vi "Actor Core.vi"(8 "error in":errorcluster, 11 "RandomDataChart in":refnum<class "MultiSubscriber.lvclass">) -> (0 "error out":errorcluster, 3 "Actor out":refnum<class "Actor.lvclass">)   [LabVIEW 2018, in "TestViewables.lvlib" / "MultiSubscriber.lvclass"]
doc: "(<B>Filename</B>: Actor Framework.lvlib:Actor.lvclass:Actor Core.vi)\n\nReceives messages to the actor, reacts to them, and initiates any error handling that may shut the actor down.\n\nDescendant classes may override this VI to append parallel tasks for the actor to complete while it handles messages. Overrides use the Call Parent Method node.\n\n<License>\nCopyright © 2017 Composed Systems, LLC | All rights reserved\nwww.composed.io\n\nAuthor: Ethan Stern <ethan.stern@composed.io>\n\nThis software is provided \"AS IS\" WITHOUT WARRANTIES, either express or implied, AND IS FOR EDUCATIONAL PURPOSES ONLY.\n</License>"
uses:
  MultiSubscriber.lvclass
  <vilib>/ActorFramework/Actor/Actor.lvclass
  MultiSubscriber Messages/Notification Msg/UpdateChart Msg.lvclass
  <vilib>/event_ctls.llb/lveventtype.ctl
  modules/mva-core/Source/SubscriptionPolicy/BasicSubscription/BasicSubscription.lvclass/BasicSubscription.ctl
  <vilib>/ActorFramework/Actor/Actor.lvclass/Actor.ctl
  <vilib>/ActorFramework/Message Enqueuer/Message Enqueuer.lvclass/Message Enqueuer.ctl
  modules/composed-transport/Source/Concrete/ActorMessageTransport/ActorMessageTransport.lvclass/ActorMessageTransport.ctl
  modules/mva-core/Source/IMediator/SubscriptionRequest/SubscriptionRequest.lvclass/SubscriptionRequest.ctl
  modules/mva-core/Source/IObserver/IObserver Messages/Subscribe Msg/Subscribe Msg.lvclass/Subscribe Msg.ctl
  MultiSubscriber.lvclass/MultiSubscriber.ctl
  modules/mva-core/Source/IMediator/SubscriptionRequest/Pack Subscription Request.vi
  modules/mva-core/Source/IObserver/IObserver Messages/Subscribe Msg/Send Subscribe.vi
  <vilib>/ActorFramework/Actor/Read Self Enqueuer.vi
  modules/composed-transport/Source/Concrete/ActorMessageTransport/Construct Actor Message Transport.vi
  <vilib>/ActorFramework/Message Enqueuer/Enqueue.vi
  <vilib>/ActorFramework/Message Enqueuer/Init from Existing Queue.vi
  <vilib>/ActorFramework/Message Enqueuer/Equals Not A Refnum.vi
  modules/mva-core/Source/SubscriptionPolicy/BasicSubscription/BasicSubscription.lvclass
  modules/mva-core/Source/IObserver/IObserver/IObserver.lvclass
  C:/Program Files (x86)/National Instruments/LabVIEW 2018/vi.lib/ActorFramework/Actor/Actor.lvclass
  modules/composed-transport/Source/Concrete/ActorMessageTransport/ActorMessageTransport.lvclass
  modules/mva-core/Source/IObserver/IObserver Messages/Subscribe Msg/Subscribe Msg.lvclass
  C:/Program Files (x86)/National Instruments/LabVIEW 2018/vi.lib/ActorFramework/Message/Message.lvclass
  <vilib>/Utility/error.llb/Error Cluster From Error Code.vi
  modules/mva-core/Source/IMediator/ISubscriptionPolicy/Open Subscription Policy.vi
  <vilib>/ActorFramework/Message Priority Queue/Priority Enqueue.vi
  <vilib>/ActorFramework/Message Enqueuer/Message Enqueuer.lvclass
  modules/mva-core/Source/IMediator/SubscriptionRequest/SubscriptionRequest.lvclass
  modules/composed-transport/Source/Concrete/ActorMessageTransport/Notification Msg/Notification Msg.lvclass
  modules/mva-viewable/Source/IViewable/IViewable/IViewable.lvclass
  modules/mva-viewable/Source/ActorEvents/IEventAggregator/IEventAggregator.lvclass
panel:
  in  "Process State":dbl
  in  "Launch Dialog":bool
  out "Cluster":T1
  in  "Random Number":dbl
  out "User Value":dbl(graph)
  # "Black Pane\nif Transparency\nis not working\nproperly"
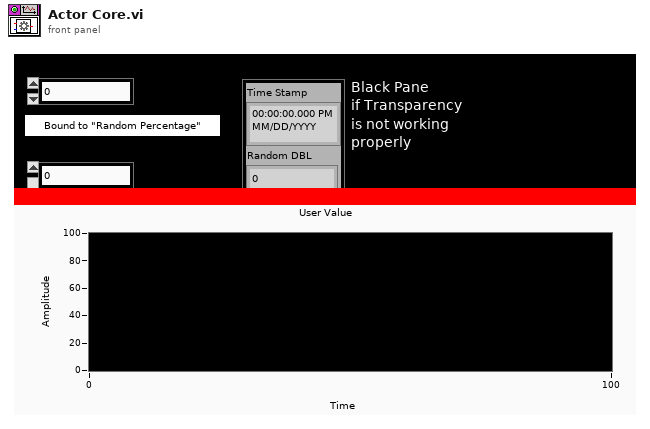
[diagram p1: front panel]
types:
  T1 = cluster{"Time Stamp":timestamp, "Random DBL":dbl}
  T2 = typedef "lveventtype.ctl" = enum32{"Null", "Timeout", "Annotation Menu Selection", "Annotation Menu Selection?", "App Instance Close", "App Instance Close?", "Autoscale Range Change", "Bookmark Info Change", "Cell Edit", "Cell Edit?", "Cursor Grab", "Cursor Grab?", "Cursor Menu Selection", "Cursor Menu Selection?", "Cursor Move", "Cursor Release", "Data Change", "Direction Change", "Display State Change", "Drag Ended", "Drag Enter", "Drag Leave", "Drag Over", "Drag Source Update", "Drag Starting", "Drag Starting?", "Drop", "Exec State Change", "Key Down", "Key Down?", "Key Repeat", "Key Repeat?", "Key Up", "Listbox Double Click", "Menu Activation?", "Menu Selection (App)", "Menu Selection? (App)", "Menu Selection (User)", "Mouse Down", "Mouse Down?", "Mouse Enter", "Mouse Leave", "Mouse Move", "Mouse Up", "Mouse Wheel", "NI Security User Change (App)", "Pane Size", "Panel Close", "Panel Close?", "Panel Resize", "Plot Attribute Change", "Scale Range Change", "Shortcut Menu Activation?", "Shortcut Menu Selection (App)", "Shortcut Menu Selection? (App)", "Shortcut Menu Selection (User)", "Tree Double Click", "Tree Drag", "Tree Drag?", "Tree Drop", "Tree Drop?", "Tree Item Close", "Tree Item Close?", "Tree Item Open", "Tree Item Open?", "User Event", "Value Change"}
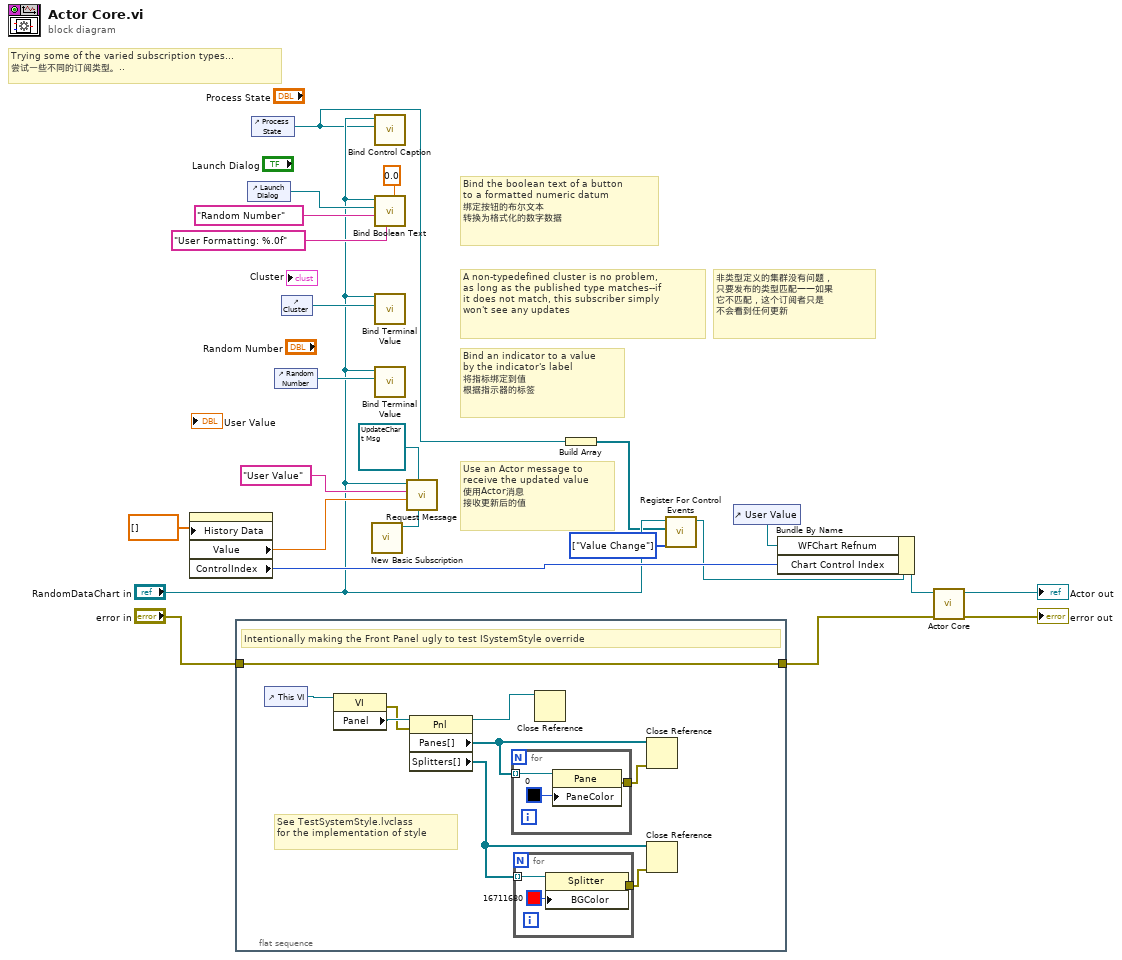
[diagram p0: block diagram]
diagram:
  w1 = T2[] [enum."Value Change"] items=["Null", "Timeout", "Annotation Menu Selection", "Annotation Menu Selection?", "App Instance Close", "App Instance Close?", "Autoscale Range Change", "Bookmark Info Change", "Cell Edit", "Cell Edit?", "Cursor Grab", "Cursor Grab?", "Cursor Menu Selection", "Cursor Menu Selection?", "Cursor Move", "Cursor Release", "Data Change", "Direction Change", "Display State Change", "Drag Ended", "Drag Enter", "Drag Leave", "Drag Over", "Drag Source Update", "Drag Starting", "Drag Starting?", "Drop", "Exec State Change", "Key Down", "Key Down?", "Key Repeat", "Key Repeat?", "Key Up", "Listbox Double Click", "Menu Activation?", "Menu Selection (App)", "Menu Selection? (App)", "Menu Selection (User)", "Mouse Down", "Mouse Down?", "Mouse Enter", "Mouse Leave", "Mouse Move", "Mouse Up", "Mouse Wheel", "NI Security User Change (App)", "Pane Size", "Panel Close", "Panel Close?", "Panel Resize", "Plot Attribute Change", "Scale Range Change", "Shortcut Menu Activation?", "Shortcut Menu Selection (App)", "Shortcut Menu Selection? (App)", "Shortcut Menu Selection (User)", "Tree Double Click", "Tree Drag", "Tree Drag?", "Tree Drop", "Tree Drop?", "Tree Item Close", "Tree Item Close?", "Tree Item Open", "Tree Item Open?", "User Event", "Value Change"] ("Registration Types")
  # "非类型定义的集群没有问题，\n只要发布的类型匹配——如果\n它不匹配，这个订阅者只是\n不会看到任何更新"
  # "Trying some of the varied subscription types...\n尝试一些不同的订阅类型。.."
  # "Bind an indicator to a value\nby the indicator's label\n将指标绑定到值\n根据指示器的标签"
  # "Bind the boolean text of a button\nto a formatted numeric datum\n绑定按钮的布尔文本\n转换为格式化的数字数据"
  # "A non-typedefined cluster is no problem,\nas long as the published type matches--if\nit does not match, this subscriber simply\nwon't see any updates"
  # "Use an Actor message to\nreceive the updated value\n使用Actor消息\n接收更新后的值"
  n1 = property on="User Value" class="WFChart (严格)"("History Data"=dbl[] []) -> ("Value"=w6:dbl, "ControlIndex"=w19:i32)  [unwired: 2 in, 2 out]
  n2 = flat-sequence {
    tunnel: "error in" -> [w26]
    tunnel: [w26] -> w8
    frame #0 {
      # "See TestSystemStyle.lvclass\nfor the implementation of style"
      # "Intentionally making the Front Panel ugly to test ISystemStyle override"
      n3 = control-ref of="This VI"() -> (w32:refnum<vi>)
      n4 = property class="VI"(reference=w32) -> (error out=w24:errorcluster, "Panel"=w31:refnum<vi>)  [unwired: 1 in, 1 out]
      n5 = property class="Pnl"(reference=w31, error in=w24) -> (reference out=w25:refnum<vi>, "Panes[]"=w28:refnum<vi>[], "Splitters[]"=w27:refnum<vi>[])  [unwired: 1 out]
      n6 = for {
        tunnel: [w37] -> w30
        tunnel: w28 -> [w36] mode=indexing
        n7 = property class="Pane"(reference=w36, "PaneColor"=u32 0) -> (error out=w37:errorcluster)  [unwired: 1 in, 1 out]
      }
      n8 = for {
        tunnel: [w34] -> w29
        tunnel: w27 -> [w33] mode=indexing
        n9 = property class="Splitter"(reference=w33, "BGColor"=u32 16711680) -> (error out=w34:errorcluster)  [unwired: 1 in, 1 out]
      }
      n10 = Close Reference(reference=w25) -> ()  [unwired: 1 in, 1 out]
      n11 = Close Reference(reference=w28, error in (no error)=w30) -> ()  [unwired: 1 out]
      n12 = Close Reference(reference=w27, error in (no error)=w29) -> ()  [unwired: 1 out]
    }
  }
  n13 = control-ref of="Launch Dialog"() -> (w10:refnum<vi>)
  n14 = control-ref of="Process State"() -> (w3:refnum<vi>)
  n15 = control-ref of="Random Number"() -> (w21:refnum<vi>)
  n16 = control-ref of="Cluster"() -> (w11:refnum<vi>)
  n17 = call "New Basic Subscription.vi"() -> ("BasicSubscription Out"=w7:refnum<class "BasicSubscription.lvclass">)  [unwired: 11 in]
  n18 = call "Bind Control Caption.vi"("Control Refnum"=w3, "IViewable in"="RandomDataChart in") -> ()  [unwired: 8 in, 2 out]
  n19 = call "Bind Boolean Text.vi"("Datum Type"=0.0, "Format String"="User Formatting: %.0f", "Datum Name (\"\"=Use Control Label)"="Random Number" ("Topic Name (Use Control Text)"), "Bool Refnum"=w10, "IViewable in"="RandomDataChart in") -> ()  [unwired: 5 in, 2 out]
  n20 = call "Bind Terminal Value.vi"("Ctl Refnum"=w11, "IViewable in"="RandomDataChart in") -> ()  [unwired: 8 in, 2 out]
  n21 = call "Bind Terminal Value.vi"("Ctl Refnum"=w21, "IViewable in"="RandomDataChart in") -> ()  [unwired: 8 in, 2 out]
  n22 = call "Request Message.vi"("Configured SubscriptionPolicy"=w7, "Desired Notification Msg"=refnum<class "UpdateChart Msg.lvclass"> refnum ("TestActors.lvlib:MultiSubscriberNotification Msg.lvclass"), "Data Type"=w6, "Datum Name"="User Value" ("Topic Name"), "IObserver in"="RandomDataChart in") -> ()  [unwired: 4 in, 3 out]
  n23 = Build Array(w3) -> (w2:refnum<vi>[])
  n24 = call "Register For Control Events.vi"("Registration Types"=w1, "Control Refnums"=w2, "IEventAggregator In"="RandomDataChart in") -> ("IEventAggregator Out"=w4:refnum<class "MultiSubscriber.lvclass">)  [unwired: 7 in, 1 out]
  n25 = control-ref of="User Value"() -> (w18:refnum<vi>)
  n26 = Bundle By Name(cluster=w4, "WFChart Refnum"=w18, "Chart Control Index"=w19) -> (w20:refnum<class "MultiSubscriber.lvclass">)
  n27 = call-parent "Actor Core.vi"("error in"=w8, "IViewable In"=w20) -> ("error out"=→"error out":errorcluster, "Actor out"=→"Actor out":refnum<class "Actor.lvclass">)  [unwired: 8 in]
